vi "Unregister and Close Sessions.vi"(8 "error in":errorcluster) -> (0 "error out":errorcluster)   [LabVIEW 2020, in "NIDmmMeasurement.lvlib"]
uses:
  NIDmmMeasurement.lvlib
  <vilib>/Plug-In SDKs/Clients/Session Management V1/Session Reservation/Session Reservation.lvclass
  <vilib>/Plug-In SDKs/Sessions/niDMM/NI Session Management niDMM.lvlib
  <vilib>/Plug-In SDKs/Clients/Session Management V1/Session Reservation/Initialize and Close Session Behavior.ctl
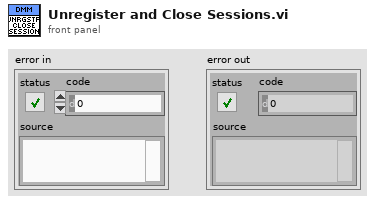
[diagram p1: front panel]
types:
  T1 = typedef "NI Session Management V1 Client.lvlib/Session Reservation.lvclass/Initialize and Close Session Behavior.ctl" = enum16{"Auto", "Initialize and Close", "Attach and Detach", "Initialize and Detach", "Attach and Close"}
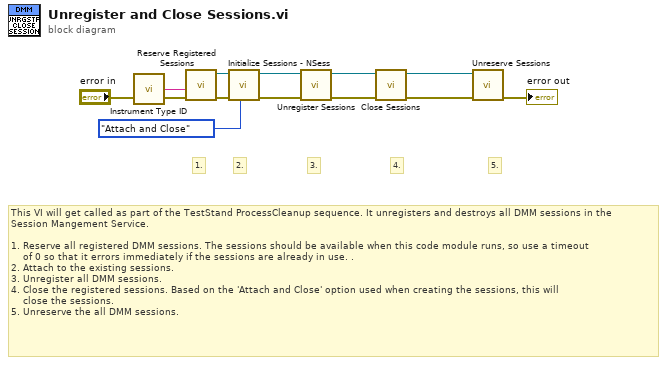
[diagram p0: block diagram]
diagram:
  # "5."
  # "4."
  # "3."
  # "2."
  # "1."
  # "This VI will get called as part of the TestStand ProcessCleanup sequence. It unregisters and destroys all DMM sessions in the\nSession Mangement Service.\n\n1. Reserve all registered DMM sessions. The sessions should be available when this code module runs, so use a timeout\n    of 0 so that it errors immediately if the sessions are already in use. .\n2. Attach to the existing sessions.\n3. Unregister all DMM sessions.\n4. Close the registered sessions. Based on the 'Attach and Close' option used when creating the sessions, this will\n    close the sessions.\n5. Unreserve the all DMM sessions."
  n1 = call <vilib>:"Instrument Type ID.vi"() -> ("instrument type id"=w7:string)  [unwired: 5 in]
  n2 = call <vilib>:"Reserve Registered Sessions.vi"("error in"="error in", "instrument type id"=w7) -> ("error out"=w9:errorcluster, "session reservation out"=w10:refnum<class "Session Reservation.lvclass">)  [unwired: 8 in]
  n3 = call <vilib>:"Initialize Sessions - NSess.vi"("initialize and close session behavior"=Initialize_and_Close_Session_Behavior."Attach and Close", "error in"=w9, "session reservation in"=w10) -> ("error out"=w5:errorcluster, "session reservation out"=w8:refnum<class "Session Reservation.lvclass">)  [unwired: 5 in, 2 out]
  n4 = call <vilib>:"Unregister Sessions.vi"("error in"=w5, "session reservation in"=w8) -> ("error out"=w4:errorcluster, "session reservation out"=w3:refnum<class "Session Reservation.lvclass">)  [unwired: 8 in]
  n5 = call <vilib>:"Close Sessions.vi"("error in"=w4, "session reservation in"=w3) -> ("error out"=w1:errorcluster, "session reservation out"=w2:refnum<class "Session Reservation.lvclass">)  [unwired: 8 in]
  n6 = call <vilib>:"Unreserve Sessions.vi"("error in"=w1, "session reservation in"=w2) -> ("error out"=→"error out":errorcluster)  [unwired: 9 in]
